vi "SaveTempData.vi"(4 "Module":string, 6 "File Handle":T1 format="%.0x", 7 "Save Data?":bool, 8 "error in (no error)":errorcluster, 10 "String":string) -> (0 "error out":errorcluster, 3 "File Handle Out":T1 format="%.0x")   [LabVIEW 2014]
uses:
  <vilib>/addons/h5labview2/base/hid_t.ctl
  <vilib>/addons/h5labview2/base/lib_path.vi
  <vilib>/addons/h5labview2/base/H5Equery.vi
  <vilib>/addons/h5labview2/dataset/H5Dwrite.llb/H5Dwrite.xnode
  <vilib>/addons/h5labview2/group/H5G.lvlib
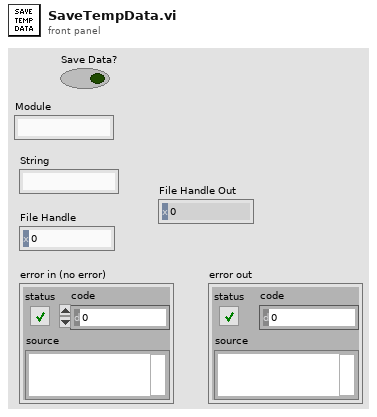
[diagram p1: front panel]
types:
  T1 = typedef "hid_t.ctl" = i32
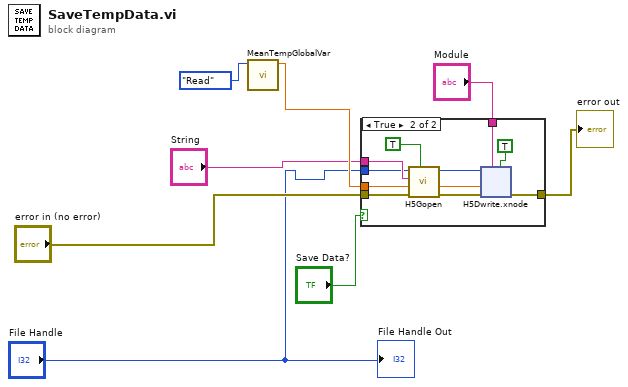
[diagram p0: block diagram]
diagram:
  n1 = call "MeanTempGlobalVar.vi"("State"=enum16{"Initialise", "Write", "Read"}."Read") -> ("Temp out"=w6:sgl)  [unwired: 10 in]
  n2 = case shown="True" "Save Data?" {
    tunnel: "error in (no error)" -> [w9 w13]
    tunnel: "File Handle" -> [_ w12]
    tunnel: "Module" -> [_ w18]
    tunnel: [w9 w17] -> w7
    tunnel: w6 -> [_ w16]
    tunnel: "String" -> [_ w15]
    frame False {
    }
    frame True {
      n3 = call <vilib>:"H5Gopen.vi"("create? (F)"=TRUE, "error in (no error)"=w13, "name"=w15, "ref in"=w12) -> ("error out"=w10:errorcluster, "group out"=w11:T1)  [unwired: 6 in]
      n4 = xnode "H5Dwrite.xnode"("replace? (F)"=TRUE, "dataset name"=w18, "error in (no error)"=w10, "data"=w16, "ref in"=w11) -> ("error out"=w17:errorcluster)  [unwired: 2 in, 2 out]
    }
  }
  "error out" <- w7
  "File Handle Out" <- "File Handle"
